vi "Parse Pirani 1.vi"(11 "Buffer in":string) -> (2 "DBL data":dbl, 3 "bytes out":string)   [LabVIEW 2019, in "PGC2D.lvlib"]
uses:
  PGC2D.lvlib
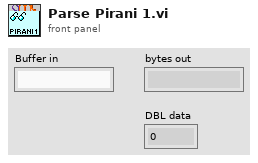
[diagram p1: front panel]
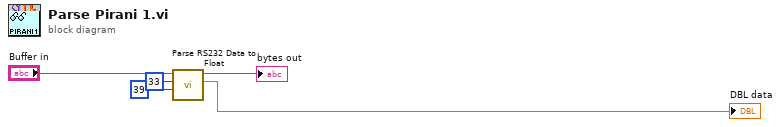
[diagram p0: block diagram]
diagram:
  n1 = call "Parse RS232 Data to Float.vi"("AML end byte"=39, "AML start byte"=33, "bytes in"="Buffer in") -> ("DBL data"=→"DBL data":dbl, "bytes out"=→"bytes out":string)  [unwired: 7 in]
